vi "contador2_global.vi"() -> ()   [LabVIEW 2017]
panel:
  in  "contador 2":u64 caption="contador 1"
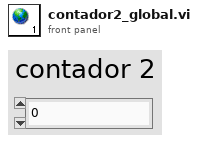
[diagram p1: front panel]
diagram:
